vi "Test Get Top Controls.vi"() -> ()   [LabVIEW 2014]
panel:
  in  "DataType":string(combo)="error"
  out "#controls":i32
  in  "vi path":path=path "C:/Users/lubo/Documents/LabView/LabVIEW-Universal-Transcriptor/Test/Example Test 1.vi"
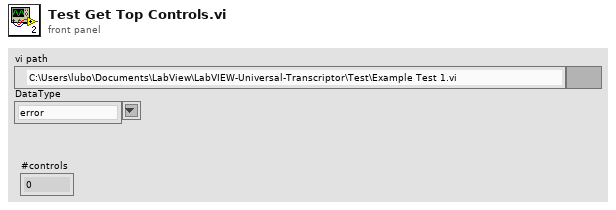
[diagram p1: front panel]
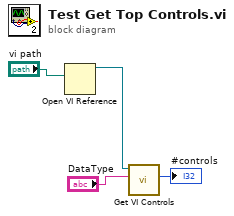
[diagram p0: block diagram]
diagram:
  n1 = Open VI Reference(vi path="vi path") -> (vi reference=w1:refnum<vi>)  [unwired: 5 in, 1 out]
  n2 = call "Get VI Controls.vi"("DataType"="DataType", "VI ref."=w1) -> ("#controls"=→"#controls":i32)  [unwired: 8 in, 1 out]
